vi "Write ip.vi"(8 "error in (no error)":errorcluster, 10 "ip":string, 11 "Motor in":refnum<class "Motor.lvclass">) -> (0 "error out":errorcluster, 3 "Motor out":refnum<class "Motor.lvclass">)   [LabVIEW 2018, in "Motor.lvclass"]
uses:
  Motor.lvclass
  Motor.lvclass/Motor.ctl
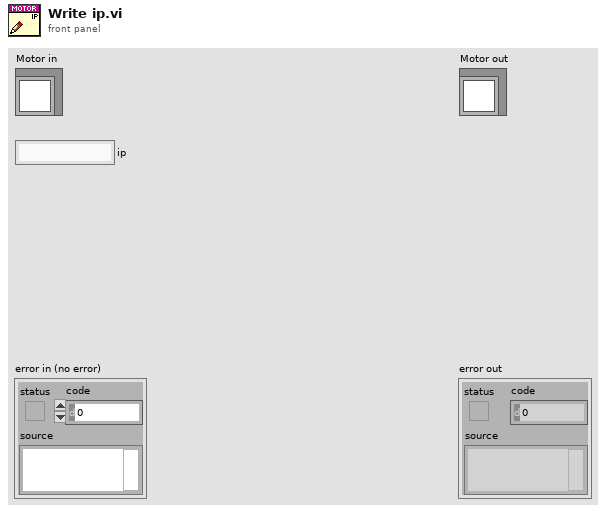
[diagram p1: front panel]
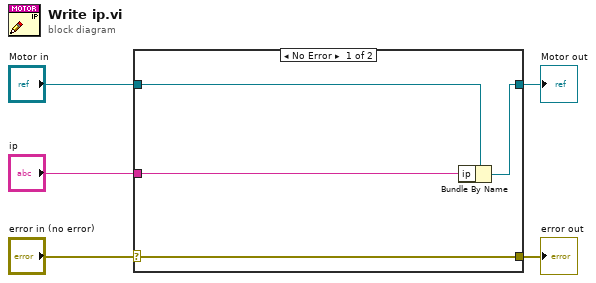
[diagram p0: block diagram]
diagram:
  n1 = case shown="No Error" "error in (no error)" {
    selector: "error in (no error)" -> [w9 w10]
    tunnel: [w9 w10] -> w4
    tunnel: [w7 w11] -> w2
    tunnel: "Motor in" -> [w8 w11]
    tunnel: "ip" -> [w6 _]
    frame No Error {
      n2 = Bundle By Name(cluster=w8, "ip"=w6) -> (w7:refnum<class "Motor.lvclass">)
    }
    frame Error {
    }
  }
  "error out" <- w4
  "Motor out" <- w2
